vi "WheelErrorGenerator.vi"() -> ()   [LabVIEW 2013]
panel:
  out "ReverseWheel":bool
  out "AngleError":dbl
  in  "stop":bool
  out "CorrectedDirection":dbl
  in  "Current Wheel Direction Reversed":bool
  in  "Current Direction":dbl(slide) min=-180.0 max=180.0 step=1.0 scale=-180.0..180.0
  in  "New Direction":dbl(slide) min=-180.0 max=180.0 step=1.0 scale=-180.0..180.0
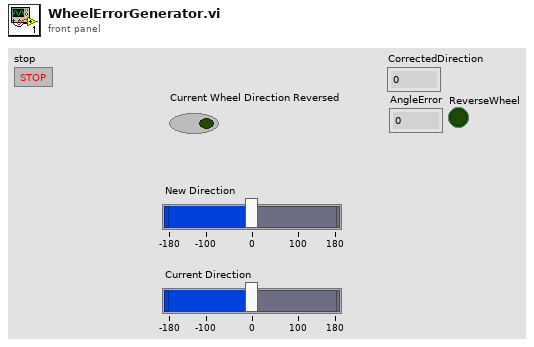
[diagram p1: front panel]
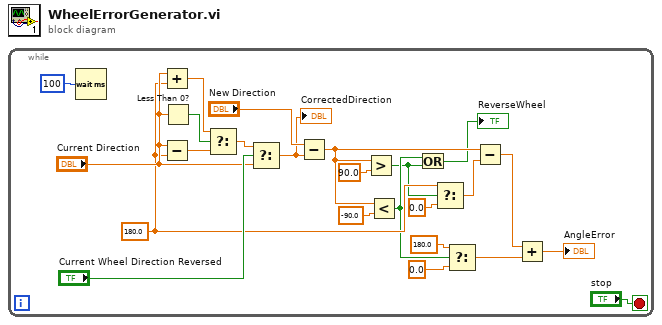
[diagram p0: block diagram]
diagram:
  n1 = while {
    stop <- "stop" stop-if-true
    w10 = 180.0 ("y")
    n2 = Wait (ms)(milliseconds to wait=u32 100) -> ()  [unwired: 1 out]
    n3 = Add(x="Current Direction", y=w10) -> (x+y=w20:dbl)
    n4 = Subtract(x="Current Direction", y=w10) -> (x-y=w19:dbl)
    n5 = Less Than 0?(x="Current Direction") -> (x < 0?=w21:bool)
    n6 = Select(t=w20, s=w21, f=w19) -> (s? t:f=w18:dbl)
    n7 = Select(t=w18, s="Current Wheel Direction Reversed", f="Current Direction") -> (s? t:f=w15:dbl)
    "CorrectedDirection" <- w15
    n8 = Subtract(x="New Direction", y=w15) -> (x-y=w9:dbl)
    n9 = Greater?(x=w9, y=90.0) -> (0:w2:bool)
    n10 = Less?(x=w9, y=-90.0) -> (x < y?=w3:bool)
    n11 = Or(x=w3, y=w2) -> (x .or. y?=→"ReverseWheel":bool)
    n12 = Select(t=w10, s=w2, f=0.0) -> (s? t:f=w12:dbl)
    n13 = Select(t=180.0, s=w3, f=0.0) -> (s? t:f=w6:dbl)
    n14 = Subtract(x=w9, y=w12) -> (x-y=w13:dbl)
    n15 = Add(x=w13, y=w6) -> (x+y=→"AngleError":dbl)
  }
